vi "Tester 2.vi"() -> ()   [LabVIEW 2017]
uses:
  Filled Text Fields Actor/Filled Text Fields Facade.ctl
  Filled Text Fields Actor/Filled Text Fields/Set Helper Text.vi
  Filled Text Fields Actor/Filled Text Fields/Set Password Display.vi
  Filled Text Fields Actor/Filled Text Fields/Filled Text Fields.lvclass
  Filled Text Fields Actor/Filled Text Fields.lvlib
panel:
  in  "Password":T1 caption="Filled String"
  in  "Login":T1 caption="Filled String"
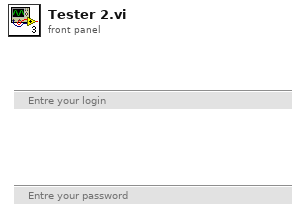
[diagram p1: front panel]
types:
  T1 = typedef "Filled Text Fields.lvlib/Filled Text Fields Facade.ctl" = cluster{"Label":string}
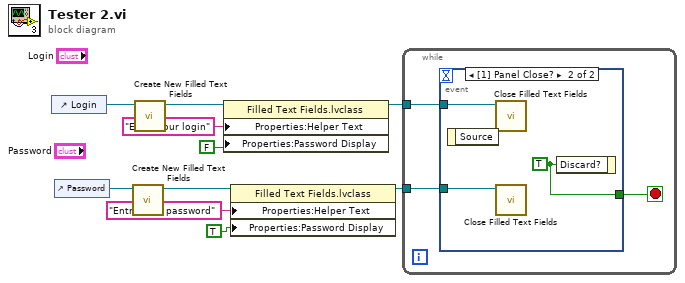
[diagram p0: block diagram]
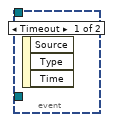
[diagram p2: hidden frame]
diagram:
  n1 = control-ref of="Login"() -> (w9:refnum<vi>)
  n2 = control-ref of="Password"() -> (w10:refnum<vi>)
  n3 = call "Create New Filled Text Fields.vi"("Filled Text Fields Ref"=w10) -> ("Filled Text Fields out"=w4:refnum<class "Filled Text Fields.lvclass">)  [unwired: 9 in, 1 out]
  n4 = call "Create New Filled Text Fields.vi"("Filled Text Fields Ref"=w9) -> ("Filled Text Fields out"=w8:refnum<class "Filled Text Fields.lvclass">)  [unwired: 9 in, 1 out]
  n5 = property class="Filled Text Fields.lvclass"(reference=w8, "Properties:Helper Text"="Entre your login" ("Helper Text"), "Properties:Password Display"=FALSE ("Password Display")) -> (reference out=w7:refnum<class "Filled Text Fields.lvclass">)  [unwired: 1 in, 1 out]
  n6 = property class="Filled Text Fields.lvclass"(reference=w4, "Properties:Helper Text"="Entre your password" ("Helper Text"), "Properties:Password Display"=TRUE ("Password Display")) -> (reference out=w3:refnum<class "Filled Text Fields.lvclass">)  [unwired: 1 in, 1 out]
  n7 = while {
    tunnel: w7 -> [w11]
    tunnel: w3 -> [w12]
    stop <- w13 stop-if-true
    n8 = event shown="[1] Panel Close?" {
      selector: _ -> [_ _]
      dyn-events: _ -> [_ _]
      timeout: _ -> [_ _]
      tunnel: [_ w16] -> w13
      tunnel: w12 -> [_ w15]
      tunnel: w11 -> [_ w14]
      event Timeout {
        n9 = event-data() -> ()  [unwired: 1 in, 3 out]
      }
      event Panel Close? {
        w16 = TRUE ("Discard?")
        n10 = event-data() -> ()  [unwired: 1 in, 1 out]
        n11 = call "Close Filled Text Fields.vi"("Filled Text Fields in"=w14) -> ()  [unwired: 10 in, 1 out]
        n12 = call "Close Filled Text Fields.vi"("Filled Text Fields in"=w15) -> ()  [unwired: 10 in, 1 out]
        n13 = event-data("Discard?"=w16) -> ()  [unwired: 1 in, 1 out]
      }
    }
  }
